vi "TestManyButtons.vi"(1 "Testable Button Array":T2(array[ring]), 2 "Buttons":T1, 3 "ButtonProfile":i32[](array[numeric])) -> (0 "Pressed? Array":bool[](array[boolean]))   [LabVIEW 2013]
uses:
  <vilib>/Rock Robotics/WPI/Joystick/WPI_JoystickButtonState.ctl
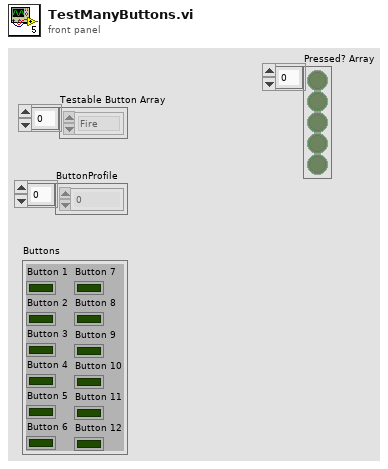
[diagram p1: front panel]
types:
  T1 = typedef "WPI_JoystickButtonState.ctl" = cluster{"Button 1":bool, "Button 2":bool, "Button 3":bool, "Button 4":bool, "Button 5":bool, "Button 6":bool, "Button 7":bool, "Button 8":bool, "Button 9":bool, "Button 10":bool, "Button 11":bool, "Button 12":bool}
  T2 = enum8{"Backward Spin WOT", "Forward Spin WOT", "Disengage WOT", "Engage WOT", "Kiddy Control", "Fire"}[]
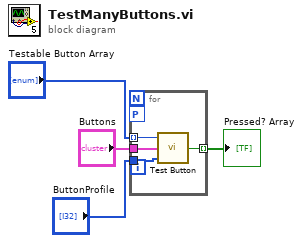
[diagram p0: block diagram]
diagram:
  n1 = for {
    tunnel: "Testable Button Array" -> [w8] mode=indexing
    tunnel: "Buttons" -> [w7]
    tunnel: "ButtonProfile" -> [w6]
    tunnel: [w5] -> w1 mode=indexing
    workers-P: _ -> [_]
    n2 = call "Test Button.vi"("ButtonProfile"=w6, "Buttons"=w7, "Button Type"=w8) -> ("Pressed?"=w5:bool)
  }
  "Pressed? Array" <- w1
